vi "Bind Insert Command Parameters.vi"(8 "Error In (no error)":errorcluster, 10 "Record":variant, 11 "SQL Statement In":refnum<class "SQL Statement.lvclass">) -> (0 "Error Out":errorcluster, 3 "SQL Statement Out":refnum<class "SQL Statement.lvclass">)   [LabVIEW 2023, in "SQLite DB Operator.lvclass"]
uses:
  SQLite DB Operator.lvclass
  <vilib>/drjdpowell/SQLite Library/SQL Statement/SQL Statement.lvclass
  DB Records/Expenses Tracker Balance/Public/Ctrls/Balance.ctl
  <vilib>/drjdpowell/SQLite Library/SQL Statement/SQL Statement.lvclass/SQL Statement.ctl
  DB Records/Expenses Tracker Category/Public/Ctrls/Category.ctl
  DB Records/Expenses Tracker Cycle/Public/Ctrls/Cycle.ctl
  DB Records/Expenses Tracker Saving Goal/Public/Ctrls/Saving Goal.ctl
  DB Records/Expenses Tracker Saving/Public/Ctrls/Saving.ctl
  DB Records/Expenses Tracker Subcategory/Public/Ctrls/Subcategory.ctl
  DB Records/Expenses Tracker Transaction/Public/Ctrls/Transaction.ctl
  <vilib>/drjdpowell/SQLite Library/SQL Statement/Bind Null.vi
  <vilib>/drjdpowell/SQLite Library/SQL Statement/Bind Timestamp (Real).vi
  <vilib>/drjdpowell/SQLite Library/SQL Statement/Bind Real.vi
  <vilib>/drjdpowell/SQLite Library/SQL Statement/Bind Text.vi
  <vilib>/drjdpowell/SQLite Library/SQL Statement/Bind Integer.vi
  <vilib>/drjdpowell/SQLite Library/SQL Statement/Error Message.vi
  DB Records/Expenses Tracker Category/Expenses Tracker Category.lvclass
  <vilib>/Utility/Data Type/NI_Data Type.lvlib
  DB Records/Expenses Tracker Transaction/Expenses Tracker Transaction.lvclass
  DB Records/Expenses Tracker Subcategory/Expenses Tracker Subcategory.lvclass
  DB Records/Expenses Tracker Balance/Expenses Tracker Balance.lvclass
  DB Records/Expenses Tracker Cycle/Expenses Tracker Cycle.lvclass
  DB Records/Expenses Tracker Saving Goal/Expenses Tracker Saving Goal.lvclass
  DB Records/Expenses Tracker Saving/Expenses Tracker Saving.lvclass
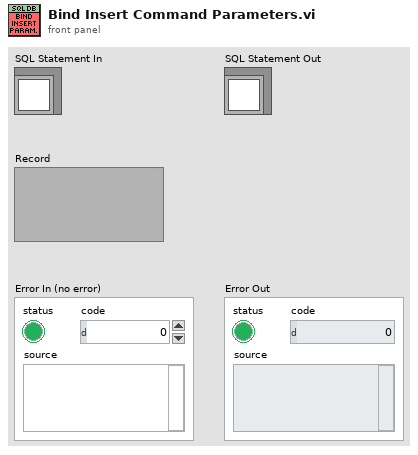
[diagram p1: front panel]
types:
  T1 = typedef "Expenses Tracker Balance.lvclass/Balance.ctl" = cluster{"ID":u8, "Value":dbl, "Last_update":timestamp}
  T2 = typedef "Expenses Tracker Category.lvclass/Category.ctl" = cluster{"ID":u32, "Name":string}
  T3 = typedef "Expenses Tracker Cycle.lvclass/Cycle.ctl" = cluster{"ID":u32, "Name":string, "Day_of_occurence":u8, "Description":string}
  T4 = typedef "Expenses Tracker Saving Goal.lvclass/Saving Goal.ctl" = cluster{"ID":u32, "Name":string, "Current_value":dbl, "Target_value":dbl, "Date_of_entry":timestamp, "Due_date":timestamp, "Last_update":timestamp, "Description":string}
  T5 = typedef "Expenses Tracker Saving.lvclass/Saving.ctl" = cluster{"ID":u32, "Saving_goal":u32, "Value":dbl, "Date_of_entry":timestamp, "Description":string}
  T6 = typedef "Expenses Tracker Subcategory.lvclass/Subcategory.ctl" = cluster{"ID":u32, "Name":string, "Category":u32}
  T7 = typedef "Expenses Tracker Transaction.lvclass/Transaction.ctl" = cluster{"ID":u32, "Name":string, "Is_income":bool, "Value":dbl, "Amount":dbl, "Total":dbl, "Date_of_entry":timestamp, "Date_of_occurence":timestamp, "Last_update":timestamp, "Category":u32, "Subcategory":u32, "Cycle":u32, "Description":string}
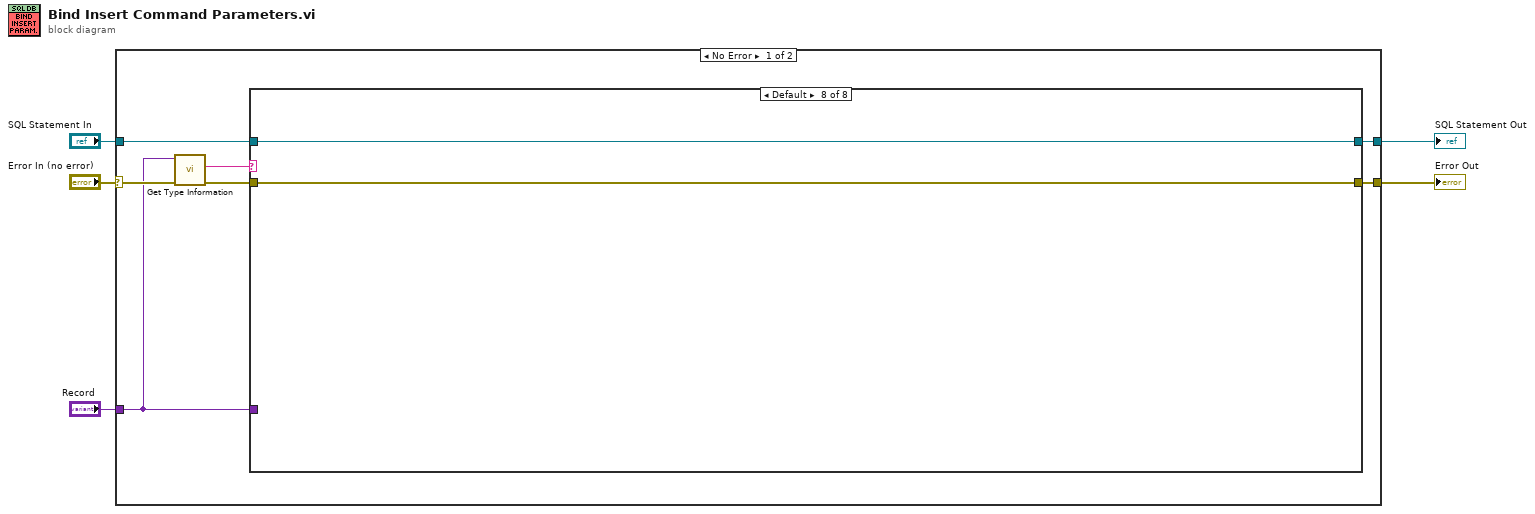
[diagram p0: block diagram]
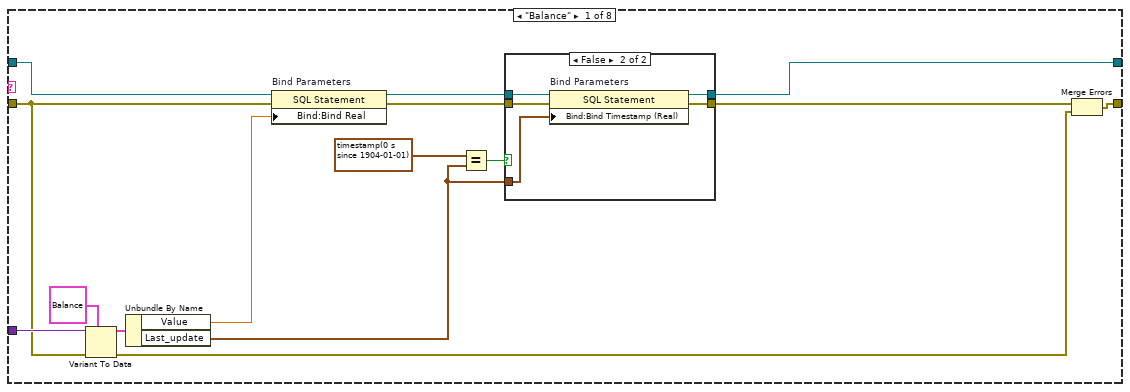
[diagram p2: hidden frame]
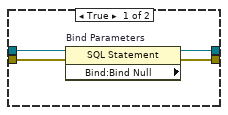
[diagram p3: hidden frame]
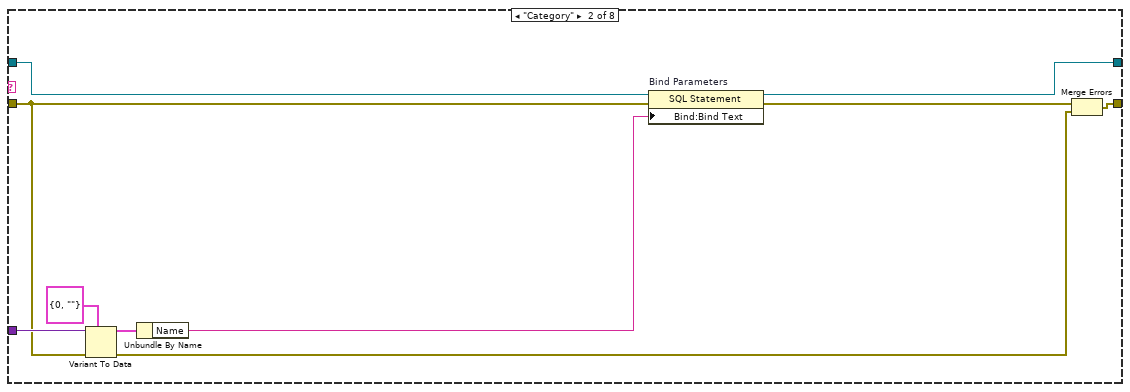
[diagram p4: hidden frame]
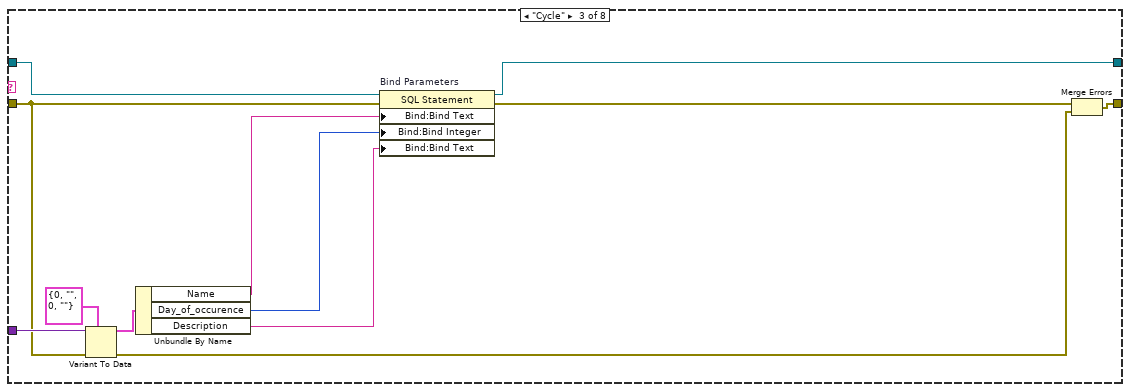
[diagram p5: hidden frame]
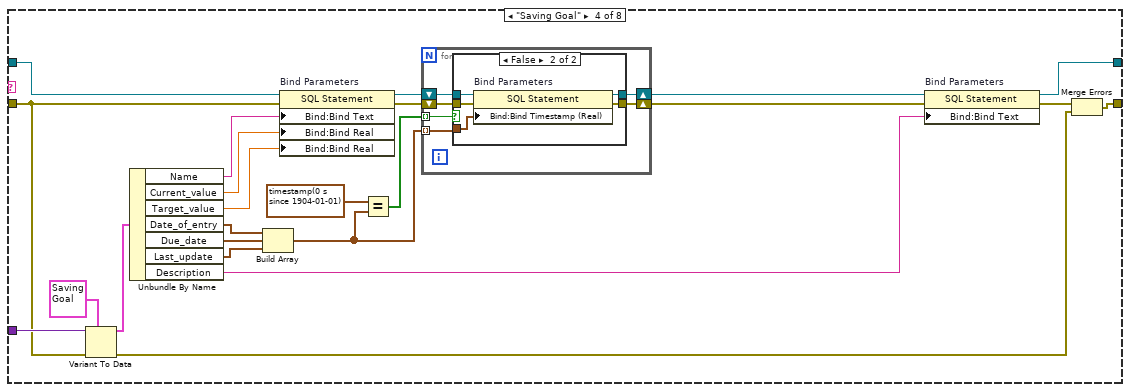
[diagram p6: hidden frame]
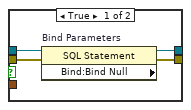
[diagram p7: hidden frame]
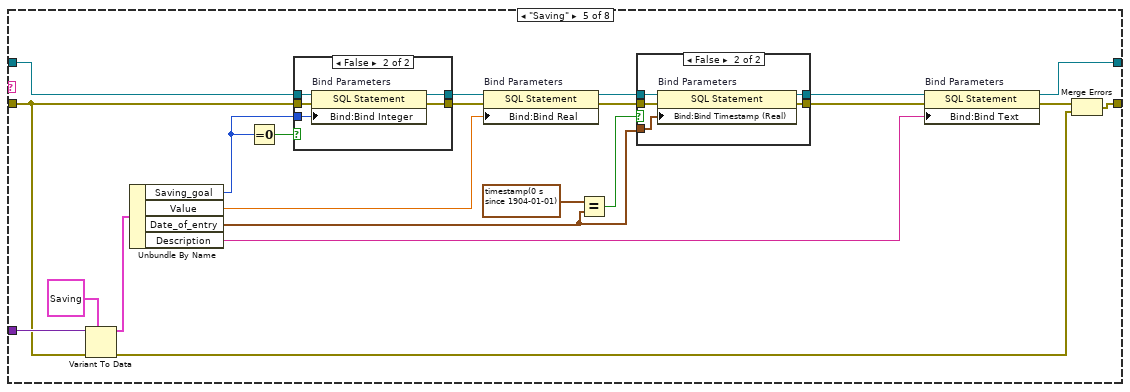
[diagram p8: hidden frame]
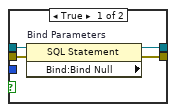
[diagram p9: hidden frame]
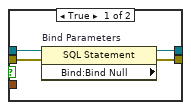
[diagram p10: hidden frame]
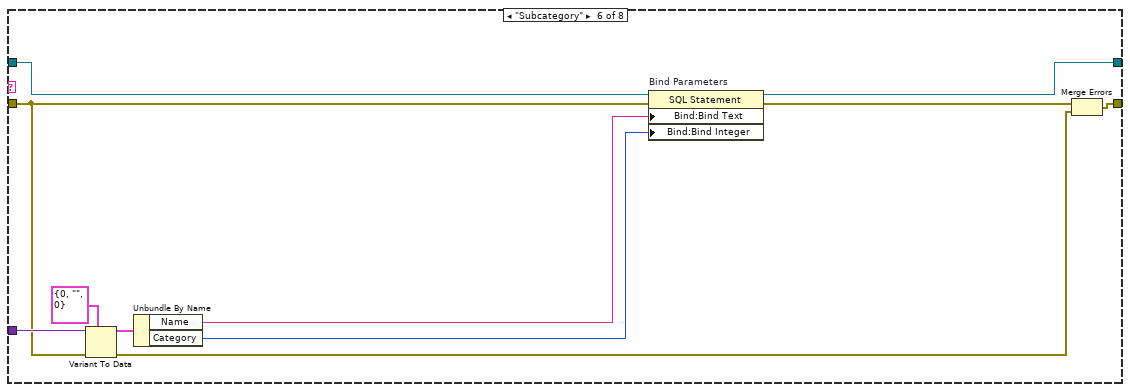
[diagram p11: hidden frame]
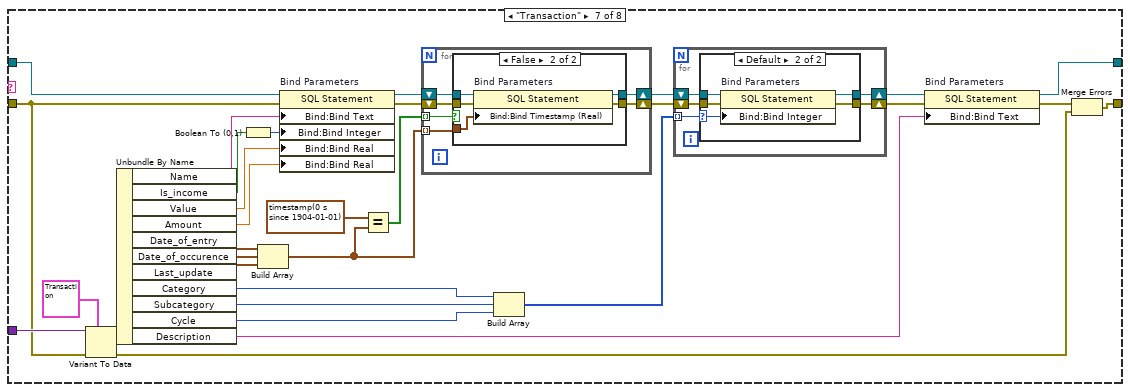
[diagram p12: hidden frame]
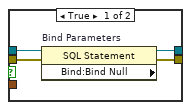
[diagram p13: hidden frame]
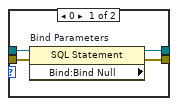
[diagram p14: hidden frame]
diagram:
  n1 = case shown="No Error" "Error In (no error)" {
    selector: "Error In (no error)" -> [w9 w210]
    tunnel: "SQL Statement In" -> [w12 w211]
    tunnel: [w11 w210] -> w4
    tunnel: [w10 w211] -> w3
    tunnel: "Record" -> [w8 _]
    frame No Error {
      n2 = call <vilib>:"Get Type Information.vi"("error in (no error)"=w9, "variant"=w8) -> ("error out"=w6:errorcluster, "name"=w7:string)  [unwired: 5 in, 3 out]
      n3 = case shown="Default" w7 {
        tunnel: w8 -> [w27 w46 w58 w81 w118 w147 w178 _]
        tunnel: [w17 w45 w49 w74 w112 w146 w165 w209] -> w10
        tunnel: [w23 w40 w54 w77 w115 w141 w174 w208] -> w11
        tunnel: w12 -> [w20 w37 w51 w72 w110 w138 w158 w209]
        tunnel: w6 -> [w21 w38 w52 w73 w111 w139 w159 w208]
        frame "Balance" {
          n4 = Variant To Data(error in=w21, type=T1 {"ID"=0, "Value"=0.0, "Last_update"=timestamp(0 s since 1904-01-01)} ("Balance"), Variant=w27) -> (data=w26:T1, error out=w22:errorcluster)
          n5 = Unbundle By Name(w26) -> ("Value"=w24:dbl, "Last_update"=w13:timestamp)
          n6 = property on="Bind Parameters" class="SQL Statement"(reference=w20, error in=w21, "Bind:Bind Real"=w24) -> (reference out=w18:refnum<class "SQL Statement.lvclass">, error out=w19:errorcluster)
          n7 = Equal?(x=timestamp(0 s since 1904-01-01), y=w13) -> (x = y?=w15:bool)
          n8 = case shown="False" w15 {
            tunnel: w19 -> [w31 w36]
            tunnel: w18 -> [w30 w35]
            tunnel: [w29 w34] -> w17
            tunnel: [w28 w33] -> w16
            tunnel: w13 -> [_ w32]
            frame True {
              n9 = property on="Bind Parameters" class="SQL Statement" props=["Bind:Bind Null"](reference=w30, error in=w31) -> (reference out=w29:refnum<class "SQL Statement.lvclass">, error out=w28:errorcluster)  [unwired: 1 out]
            }
            frame False {
              n10 = property on="Bind Parameters" class="SQL Statement"(reference=w35, error in=w36, "Bind:Bind Timestamp (Real)"=w32) -> (reference out=w34:refnum<class "SQL Statement.lvclass">, error out=w33:errorcluster)
            }
          }
          n11 = Merge Errors(w16, w22) -> (w23:errorcluster)
        }
        frame "Category" {
          n12 = Variant To Data(error in=w38, type=T2 {"ID"=0, "Name"=""} ("Category"), Variant=w46) -> (data=w43:T2, error out=w39:errorcluster)
          n13 = Unbundle By Name(w43) -> ("Name"=w41:string)
          n14 = property on="Bind Parameters" class="SQL Statement"(reference=w37, error in=w38, "Bind:Bind Text"=w41) -> (reference out=w45:refnum<class "SQL Statement.lvclass">, error out=w44:errorcluster)
          n15 = Merge Errors(w44, w39) -> (w40:errorcluster)
        }
        frame "Cycle" {
          n16 = Variant To Data(error in=w52, type=T3 {"ID"=0, "Name"="", "Day_of_occurence"=0, "Description"=""} ("Cycle"), Variant=w58) -> (data=w57:T3, error out=w53:errorcluster)
          n17 = Unbundle By Name(w57) -> ("Name"=w55:string, "Day_of_occurence"=w48:u8, "Description"=w47:string)
          n18 = property on="Bind Parameters" class="SQL Statement"(reference=w51, error in=w52, "Bind:Bind Text"=w55, "Bind:Bind Integer"=w48, "Bind:Bind Text"=w47) -> (reference out=w49:refnum<class "SQL Statement.lvclass">, error out=w50:errorcluster)
          n19 = Merge Errors(w50, w53) -> (w54:errorcluster)
        }
        frame "Saving Goal" {
          n20 = Variant To Data(error in=w73, type=T4 {"ID"=0, "Name"="", "Current_value"=0.0, "Target_value"=0.0, "Date_of_entry"=timestamp(0 s since 1904-01-01), "Due_date"=timestamp(0 s since 1904-01-01), "Last_update"=timestamp(0 s since 1904-01-01), "Description"=""} ("Saving Goal"), Variant=w81) -> (data=w80:T4, error out=w76:errorcluster)
          n21 = Unbundle By Name(w80) -> ("Name"=w78:string, "Current_value"=w64:dbl, "Target_value"=w63:dbl, "Date_of_entry"=w62:timestamp, "Due_date"=w61:timestamp, "Last_update"=w60:timestamp, "Description"=w59:string)
          n22 = Build Array(w62, w61, w60) -> (w65:timestamp[])
          n23 = property on="Bind Parameters" class="SQL Statement"(reference=w72, error in=w73, "Bind:Bind Text"=w78, "Bind:Bind Real"=w64, "Bind:Bind Real"=w63) -> (reference out=w69:refnum<class "SQL Statement.lvclass">, error out=w68:errorcluster)
          n24 = Equal?(x=timestamp(0 s since 1904-01-01), y=w65) -> (x = y?=w66:bool[])
          n25 = for {
            shift-right: [w84] -> w71
            shift-left: w68 -> [w87]
            shift-right: [w85] -> w70
            shift-left: w69 -> [w86]
            tunnel: w66 -> [w83] mode=indexing
            tunnel: w65 -> [w82] mode=indexing
            n26 = case shown="False" w83 {
              tunnel: w87 -> [w91 w96]
              tunnel: w86 -> [w90 w95]
              tunnel: [w89 w94] -> w85
              tunnel: [w88 w93] -> w84
              tunnel: w82 -> [_ w92]
              frame True {
                n27 = property on="Bind Parameters" class="SQL Statement" props=["Bind:Bind Null"](reference=w90, error in=w91) -> (reference out=w89:refnum<class "SQL Statement.lvclass">, error out=w88:errorcluster)  [unwired: 1 out]
              }
              frame False {
                n28 = property on="Bind Parameters" class="SQL Statement"(reference=w95, error in=w96, "Bind:Bind Timestamp (Real)"=w92) -> (reference out=w94:refnum<class "SQL Statement.lvclass">, error out=w93:errorcluster)
              }
            }
          }
          n29 = property on="Bind Parameters" class="SQL Statement"(reference=w70, error in=w71, "Bind:Bind Text"=w59) -> (reference out=w74:refnum<class "SQL Statement.lvclass">, error out=w75:errorcluster)
          n30 = Merge Errors(w75, w76) -> (w77:errorcluster)
        }
        frame "Saving" {
          n31 = Variant To Data(error in=w111, type=T5 {"ID"=0, "Saving_goal"=0, "Value"=0.0, "Date_of_entry"=timestamp(0 s since 1904-01-01), "Description"=""} ("Saving"), Variant=w118) -> (data=w117:T5, error out=w114:errorcluster)
          n32 = Unbundle By Name(w117) -> ("Saving_goal"=w97:u32, "Value"=w99:dbl, "Date_of_entry"=w104:timestamp, "Description"=w105:string)
          n33 = Equal To 0?(x=w97) -> (x = 0?=w98:bool)
          n34 = case shown="False" w98 {
            tunnel: w97 -> [_ w127]
            tunnel: w111 -> [w122 w126]
            tunnel: w110 -> [w121 w125]
            tunnel: [w120 w124] -> w103
            tunnel: [w119 w123] -> w102
            frame True {
              n35 = property on="Bind Parameters" class="SQL Statement" props=["Bind:Bind Null"](reference=w121, error in=w122) -> (reference out=w120:refnum<class "SQL Statement.lvclass">, error out=w119:errorcluster)  [unwired: 1 out]
            }
            frame False {
              n36 = property on="Bind Parameters" class="SQL Statement"(reference=w125, error in=w126, "Bind:Bind Integer"=w127) -> (reference out=w124:refnum<class "SQL Statement.lvclass">, error out=w123:errorcluster)
            }
          }
          n37 = property on="Bind Parameters" class="SQL Statement"(reference=w103, error in=w102, "Bind:Bind Real"=w99) -> (reference out=w100:refnum<class "SQL Statement.lvclass">, error out=w101:errorcluster)
          n38 = Equal?(x=timestamp(0 s since 1904-01-01), y=w104) -> (x = y?=w106:bool)
          n39 = case shown="False" w106 {
            tunnel: w101 -> [w131 w136]
            tunnel: w100 -> [w130 w135]
            tunnel: [w129 w134] -> w108
            tunnel: [w128 w133] -> w109
            tunnel: w104 -> [_ w132]
            frame True {
              n40 = property on="Bind Parameters" class="SQL Statement" props=["Bind:Bind Null"](reference=w130, error in=w131) -> (reference out=w129:refnum<class "SQL Statement.lvclass">, error out=w128:errorcluster)  [unwired: 1 out]
            }
            frame False {
              n41 = property on="Bind Parameters" class="SQL Statement"(reference=w135, error in=w136, "Bind:Bind Timestamp (Real)"=w132) -> (reference out=w134:refnum<class "SQL Statement.lvclass">, error out=w133:errorcluster)
            }
          }
          n42 = property on="Bind Parameters" class="SQL Statement"(reference=w108, error in=w109, "Bind:Bind Text"=w105) -> (reference out=w112:refnum<class "SQL Statement.lvclass">, error out=w113:errorcluster)
          n43 = Merge Errors(w113, w114) -> (w115:errorcluster)
        }
        frame "Subcategory" {
          n44 = Variant To Data(error in=w139, type=T6 {"ID"=0, "Name"="", "Category"=0} ("Subcategory"), Variant=w147) -> (data=w144:T6, error out=w140:errorcluster)
          n45 = Unbundle By Name(w144) -> ("Name"=w142:string, "Category"=w137:u32)
          n46 = property on="Bind Parameters" class="SQL Statement"(reference=w138, error in=w139, "Bind:Bind Text"=w142, "Bind:Bind Integer"=w137) -> (reference out=w146:refnum<class "SQL Statement.lvclass">, error out=w145:errorcluster)
          n47 = Merge Errors(w145, w140) -> (w141:errorcluster)
        }
        frame "Transaction" {
          n48 = Variant To Data(error in=w159, type=T7 {"ID"=0, "Name"="", "Is_income"=FALSE, "Value"=0.0, "Amount"=0.0, "Total"=0.0, "Date_of_entry"=timestamp(0 s since 1904-01-01), "Date_of_occurence"=timestamp(0 s since 1904-01-01), "Last_update"=timestamp(0 s since 1904-01-01), "Category"=0, "Subcategory"=0, "Cycle"=0, "Description"=""} ("Transaction"), Variant=w178) -> (data=w177:T7, error out=w173:errorcluster)
          n49 = Unbundle By Name(w177) -> ("Name"=w175:string, "Is_income"=w170:bool, "Value"=w171:dbl, "Amount"=w172:dbl, "Date_of_entry"=w153:timestamp, "Date_of_occurence"=w152:timestamp, "Last_update"=w151:timestamp, "Category"=w163:u32, "Subcategory"=w162:u32, "Cycle"=w161:u32, "Description"=w164:string)
          n50 = Boolean To (0,1)(Boolean=w170) -> (0, 1=w169:i16)
          n51 = Build Array(w153, w152, w151) -> (w148:timestamp[])
          n52 = property on="Bind Parameters" class="SQL Statement"(reference=w158, error in=w159, "Bind:Bind Text"=w175, "Bind:Bind Integer"=w169, "Bind:Bind Real"=w171, "Bind:Bind Real"=w172) -> (reference out=w155:refnum<class "SQL Statement.lvclass">, error out=w154:errorcluster)
          n53 = Equal?(x=timestamp(0 s since 1904-01-01), y=w148) -> (x = y?=w149:bool[])
          n54 = for {
            shift-right: [w181] -> w157
            shift-left: w154 -> [w184]
            shift-right: [w182] -> w156
            shift-left: w155 -> [w183]
            tunnel: w149 -> [w180] mode=indexing
            tunnel: w148 -> [w179] mode=indexing
            n55 = case shown="False" w180 {
              tunnel: w184 -> [w188 w193]
              tunnel: w183 -> [w187 w192]
              tunnel: [w186 w191] -> w182
              tunnel: [w185 w190] -> w181
              tunnel: w179 -> [_ w189]
              frame True {
                n56 = property on="Bind Parameters" class="SQL Statement" props=["Bind:Bind Null"](reference=w187, error in=w188) -> (reference out=w186:refnum<class "SQL Statement.lvclass">, error out=w185:errorcluster)  [unwired: 1 out]
              }
              frame False {
                n57 = property on="Bind Parameters" class="SQL Statement"(reference=w192, error in=w193, "Bind:Bind Timestamp (Real)"=w189) -> (reference out=w191:refnum<class "SQL Statement.lvclass">, error out=w190:errorcluster)
              }
            }
          }
          n58 = Build Array(w163, w162, w161) -> (w160:u32[])
          n59 = for {
            shift-right: [w195] -> w167
            shift-left: w157 -> [w198]
            shift-right: [w196] -> w168
            shift-left: w156 -> [w197]
            tunnel: w160 -> [w194] mode=indexing
            n60 = case shown="Default" w194 {
              selector: w194 -> [_ w203]
              tunnel: w198 -> [w202 w207]
              tunnel: w197 -> [w201 w206]
              tunnel: [w200 w205] -> w196
              tunnel: [w199 w204] -> w195
              frame 0 {
                n61 = property on="Bind Parameters" class="SQL Statement" props=["Bind:Bind Null"](reference=w201, error in=w202) -> (reference out=w200:refnum<class "SQL Statement.lvclass">, error out=w199:errorcluster)  [unwired: 1 out]
              }
              frame Default {
                n62 = property on="Bind Parameters" class="SQL Statement"(reference=w206, error in=w207, "Bind:Bind Integer"=w203) -> (reference out=w205:refnum<class "SQL Statement.lvclass">, error out=w204:errorcluster)
              }
            }
          }
          n63 = property on="Bind Parameters" class="SQL Statement"(reference=w168, error in=w167, "Bind:Bind Text"=w164) -> (reference out=w165:refnum<class "SQL Statement.lvclass">, error out=w166:errorcluster)
          n64 = Merge Errors(w166, w173) -> (w174:errorcluster)
        }
        frame Default {
        }
      }
    }
    frame Error {
    }
  }
  "Error Out" <- w4
  "SQL Statement Out" <- w3
